vi "Delay_ms.vi"(8 "error in (no error)":errorcluster, 11 "IN":T1={"step name 1"="", "updata 2"="1000", "limitdata 3"="", "load vi name 4"="", "parameter 5"=""}) -> (0 "error out":errorcluster, 3 "Cluster":T2)   [LabVIEW 2013]
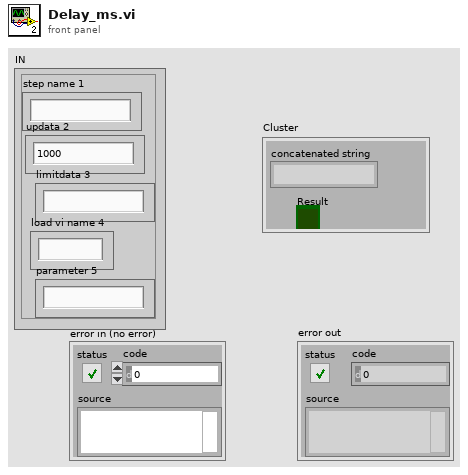
[diagram p1: front panel]
types:
  T1 = cluster{"step name 1":string, "updata 2":string, "limitdata 3":string, "load vi name 4":string, "parameter 5":string}
  T2 = cluster{"concatenated string":string, "Result":bool}
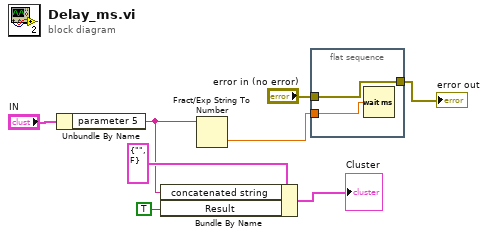
[diagram p0: block diagram]
diagram:
  n1 = Unbundle By Name("IN") -> ("parameter 5"=w3:string)
  n2 = Bundle By Name(cluster=T2 {"concatenated string"="", "Result"=FALSE} ("Cluster"), "concatenated string"=w3, "Result"=TRUE) -> (→"Cluster":T2)
  n3 = Fract/Exp String To Number(string=w3) -> (number=w4:dbl)  [unwired: 3 in, 1 out]
  n4 = flat-sequence {
    tunnel: "error in (no error)" -> [w9]
    tunnel: w4 -> [w10]
    tunnel: [w9] -> w2
    frame #0 {
      n5 = Wait (ms)(milliseconds to wait=w10) -> ()  [unwired: 1 out]
    }
  }
  "error out" <- w2
